vi "DivideAreaGen.vi"(6 "WidthDivider":i32=1, 7 "HeightDivider":i32=1, 8 "ErrorIn(No Error)":errorcluster caption="entrée d'erreur (pas d'erreur)", 9 "Position":T2, 10 "Limites":T1) -> (0 "sortie d'erreur":errorcluster, 1 "PositionsOut":T2[](array[typedef]), 2 "LimitsOut":T1)   [LabVIEW 2019]
uses:
  <vilib>/Utility/miscctls.llb/LVBoundsTypeDef.ctl
  <vilib>/Utility/miscctls.llb/LVPositionTypeDef.ctl
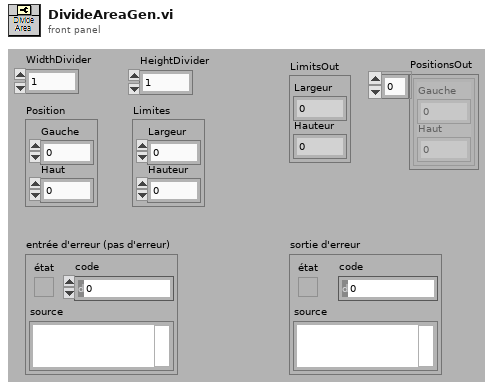
[diagram p1: front panel]
types:
  T1 = typedef "LVBoundsTypeDef.ctl" = cluster{"Width":u32, "Height":u32}
  T2 = typedef "LVPositionTypeDef.ctl" = cluster{"Left":i32, "Top":i32}
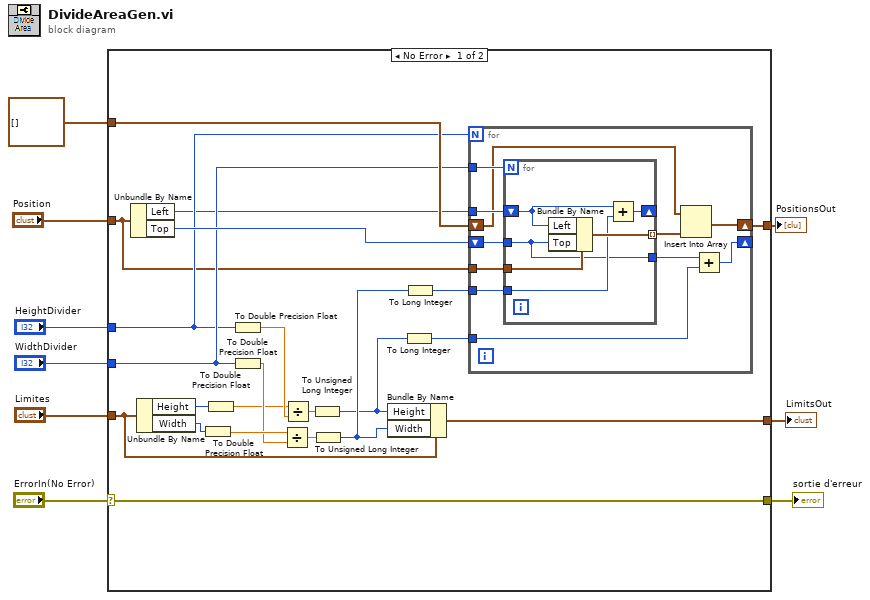
[diagram p0: block diagram]
diagram:
  n1 = case shown="No Error" "ErrorIn(No Error)" {
    selector: "ErrorIn(No Error)" -> [w12 w49]
    tunnel: [w31 _] -> w9
    tunnel: T2[] [] -> [w30 _]
    tunnel: [w29 _] -> w7
    tunnel: "WidthDivider" -> [w25 _]
    tunnel: "HeightDivider" -> [w24 _]
    tunnel: "Position" -> [w22 _]
    tunnel: "Limites" -> [w13 _]
    tunnel: [w12 w49] -> w1
    frame No Error {
      n2 = Unbundle By Name(w22) -> ("Left"=w23:i32, "Top"=w27:i32)
      n3 = Unbundle By Name(w13) -> ("Height"=w16:u32, "Width"=w20:u32)
      n4 = To Double Precision Float(number=w20) -> (double precision float=w21:dbl)
      n5 = To Double Precision Float(number=w16) -> (double precision float=w14:dbl)
      n6 = To Double Precision Float(number=w24) -> (double precision float=w15:dbl)
      n7 = To Double Precision Float(number=w25) -> (double precision float=w19:dbl)
      n8 = Divide(x=w21, y=w19) -> (x/y=w18:dbl)
      n9 = Divide(x=w14, y=w15) -> (x/y=w17:dbl)
      n10 = To Unsigned Long Integer(number=w17) -> (unsigned 32bit integer=w10:u32)
      n11 = To Unsigned Long Integer(number=w18) -> (unsigned 32bit integer=w11:u32)
      n12 = Bundle By Name(cluster=w13, "Height"=w10, "Width"=w11) -> (w31:T1)
      n13 = To Long Integer(number=w10) -> (32bit integer=w28:i32)
      n14 = To Long Integer(number=w11) -> (32bit integer=w26:i32)
      n15 = for {
        N: w24 -> [_]
        tunnel: w22 -> [w42]
        tunnel: w23 -> [w41]
        tunnel: w25 -> [w40]
        tunnel: w26 -> [w39]
        shift-right: [w37] -> _
        shift-left: w27 -> [w38]
        tunnel: w28 -> [w35]
        shift-right: [w34] -> w29
        shift-left: w30 -> [w32]
        n16 = for {
          N: w40 -> [_]
          tunnel: w42 -> [w48]
          shift-right: [w44] -> _
          shift-left: w41 -> [w46]
          tunnel: [w47] -> w33 mode=indexing
          tunnel: w39 -> [w45]
          tunnel: w38 -> [w43]
          tunnel: [w43] -> w36
          n17 = Bundle By Name(cluster=w48, "Left"=w46, "Top"=w43) -> (w47:T2)
          n18 = Add(x=w46, y=w45) -> (x+y=w44:i32)
        }
        n19 = Insert Into Array(array=w32, new element=w33) -> (w34:T2[])  [unwired: 1 in]
        n20 = Add(x=w36, y=w35) -> (x+y=w37:i32)
      }
    }
    frame Error {
    }
  }
  "sortie d'erreur" <- w1
  "PositionsOut" <- w7
  "LimitsOut" <- w9
